vi "FlatToRichni_measurementlink_measurement_v2_GetMetadataResponse.vi"(5 "OutputClusterType":T1, 11 "InputCluster":T11) -> (3 "OutputCluster":T1)   [LabVIEW 2021, in "Measurement Service Client V2.lvlib"]
uses:
  Measurement Service Client V2.lvlib
  ni_measurementlink_measurement_v2_GetMetadataResponse_Flat.ctl
  ni_measurementlink_measurement_v2_MeasurementDetails_Flat.ctl
  ni_measurementlink_measurement_v2_MeasurementSignature_Flat.ctl
  ni_measurementlink_measurement_v2_ConfigurationParameter_Flat.ctl
  google_protobuf_Field_Kind.ctl
  ni_measurementlink_measurement_v2_ConfigurationParameter_AnnotationsEntry_Flat.ctl
  google_protobuf_Any_Flat.ctl
  ni_measurementlink_measurement_v2_Output_Flat.ctl
  ni_measurementlink_measurement_v2_Output_AnnotationsEntry_Flat.ctl
  ni_measurementlink_measurement_v2_UserInterfaceDetails_Flat.ctl
  ni_measurementlink_measurement_v2_GetMetadataResponse.ctl
  ni_measurementlink_measurement_v2_MeasurementDetails.ctl
  ni_measurementlink_measurement_v2_MeasurementSignature.ctl
  ni_measurementlink_measurement_v2_ConfigurationParameter.ctl
  ni_measurementlink_measurement_v2_ConfigurationParameter_AnnotationsEntry.ctl
  google_protobuf_Any.ctl
  ni_measurementlink_measurement_v2_Output.ctl
  ni_measurementlink_measurement_v2_Output_AnnotationsEntry.ctl
  ni_measurementlink_measurement_v2_UserInterfaceDetails.ctl
  FlatToRichni_measurementlink_measurement_v2_ConfigurationParameter.vi
  FlatToRichgoogle_protobuf_Any.vi
  FlatToRichni_measurementlink_measurement_v2_Output.vi
  FlatToRichni_measurementlink_measurement_v2_ConfigurationParameter_AnnotationsEntry.vi
  FlatToRichni_measurementlink_measurement_v2_Output_AnnotationsEntry.vi
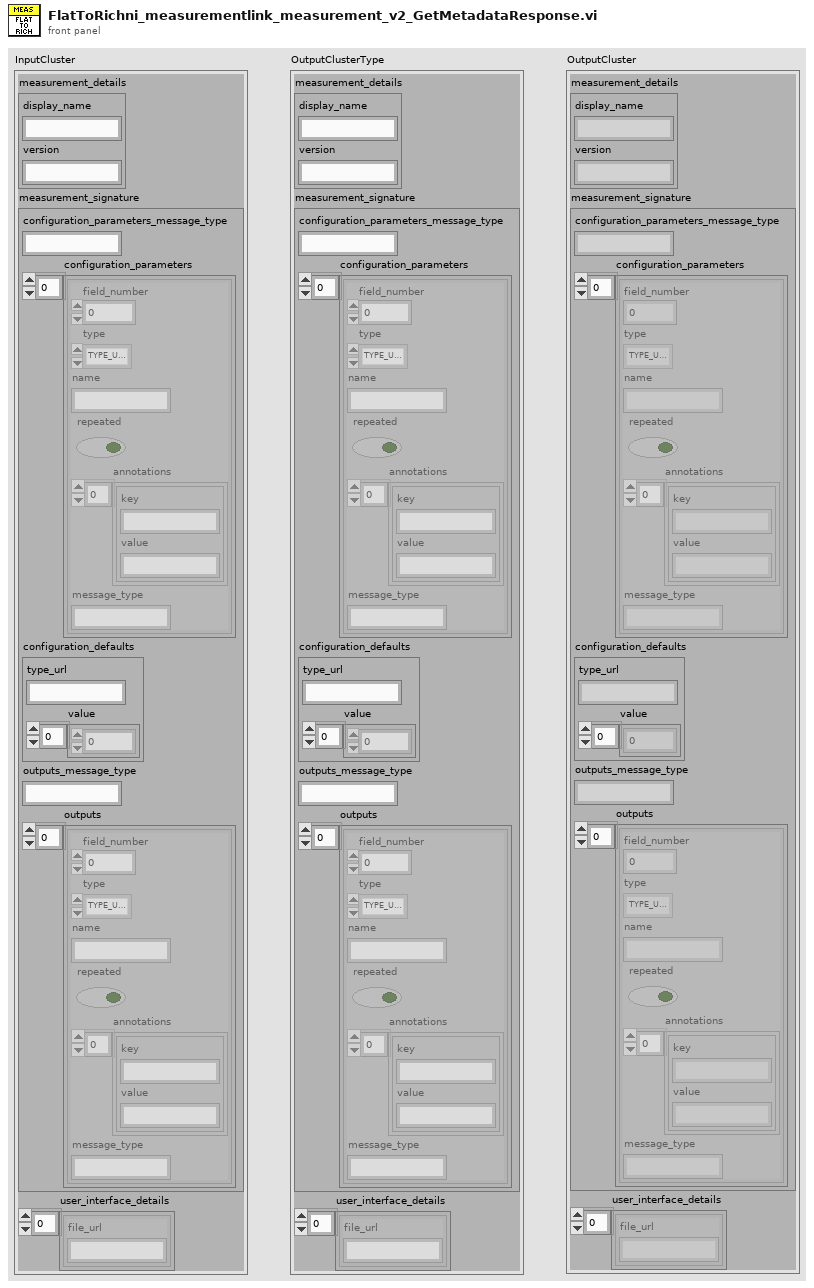
[diagram p1: front panel]
types:
  T1 = typedef "Measurement Service Client V2.lvlib/ni_measurementlink_measurement_v2_GetMetadataResponse.ctl" = cluster{"measurement_details":T2, "measurement_signature":T3, "user_interface_details":T10[]}
  T2 = typedef "Measurement Service Client V2.lvlib/ni_measurementlink_measurement_v2_MeasurementDetails.ctl" = cluster{"display_name":string, "version":string}
  T3 = typedef "Measurement Service Client V2.lvlib/ni_measurementlink_measurement_v2_MeasurementSignature.ctl" = cluster{"configuration_parameters_message_type":string, "configuration_parameters":T4[], "configuration_defaults":T7, "outputs_message_type":string, "outputs":T8[]}
  T4 = typedef "Measurement Service Client V2.lvlib/ni_measurementlink_measurement_v2_ConfigurationParameter.ctl" = cluster{"field_number":i32, "type":T5, "name":string, "repeated":bool, "annotations":T6[], "message_type":string}
  T5 = typedef "Measurement Service Client V2.lvlib/google_protobuf_Field_Kind.ctl" = enum32{"TYPE_UNKNOWN", "TYPE_DOUBLE", "TYPE_FLOAT", "TYPE_INT64", "TYPE_UINT64", "TYPE_INT32", "TYPE_FIXED64", "TYPE_FIXED32", "TYPE_BOOL", "TYPE_STRING", "TYPE_GROUP", "TYPE_MESSAGE", "TYPE_BYTES", "TYPE_UINT32", "TYPE_ENUM", "TYPE_SFIXED32", "TYPE_SFIXED64", "TYPE_SINT32", "TYPE_SINT64"}
  T6 = typedef "Measurement Service Client V2.lvlib/ni_measurementlink_measurement_v2_ConfigurationParameter_AnnotationsEntry.ctl" = cluster{"key":string, "value":string}
  T7 = typedef "Measurement Service Client V2.lvlib/google_protobuf_Any.ctl" = cluster{"type_url":string, "value":u8[]}
  T8 = typedef "Measurement Service Client V2.lvlib/ni_measurementlink_measurement_v2_Output.ctl" = cluster{"field_number":i32, "type":T5, "name":string, "repeated":bool, "annotations":T9[], "message_type":string}
  T9 = typedef "Measurement Service Client V2.lvlib/ni_measurementlink_measurement_v2_Output_AnnotationsEntry.ctl" = cluster{"key":string, "value":string}
  T10 = typedef "Measurement Service Client V2.lvlib/ni_measurementlink_measurement_v2_UserInterfaceDetails.ctl" = cluster{"file_url":string}
  T11 = typedef "Measurement Service Client V2.lvlib/ni_measurementlink_measurement_v2_GetMetadataResponse_Flat.ctl" = cluster{"measurement_details":T12, "measurement_signature":T13, "user_interface_details":T19[]}
  T12 = typedef "Measurement Service Client V2.lvlib/ni_measurementlink_measurement_v2_MeasurementDetails_Flat.ctl" = cluster{"display_name":string, "version":string}
  T13 = typedef "Measurement Service Client V2.lvlib/ni_measurementlink_measurement_v2_MeasurementSignature_Flat.ctl" = cluster{"configuration_parameters_message_type":string, "configuration_parameters":T14[], "configuration_defaults":T16, "outputs_message_type":string, "outputs":T17[]}
  T14 = typedef "Measurement Service Client V2.lvlib/ni_measurementlink_measurement_v2_ConfigurationParameter_Flat.ctl" = cluster{"field_number":i32, "type":T5, "name":string, "repeated":bool, "annotations":T15[], "message_type":string}
  T15 = typedef "Measurement Service Client V2.lvlib/ni_measurementlink_measurement_v2_ConfigurationParameter_AnnotationsEntry_Flat.ctl" = cluster{"key":string, "value":string}
  T16 = typedef "Measurement Service Client V2.lvlib/google_protobuf_Any_Flat.ctl" = cluster{"type_url":string, "value":u8[]}
  T17 = typedef "Measurement Service Client V2.lvlib/ni_measurementlink_measurement_v2_Output_Flat.ctl" = cluster{"field_number":i32, "type":T5, "name":string, "repeated":bool, "annotations":T18[], "message_type":string}
  T18 = typedef "Measurement Service Client V2.lvlib/ni_measurementlink_measurement_v2_Output_AnnotationsEntry_Flat.ctl" = cluster{"key":string, "value":string}
  T19 = typedef "Measurement Service Client V2.lvlib/ni_measurementlink_measurement_v2_UserInterfaceDetails_Flat.ctl" = cluster{"file_url":string}
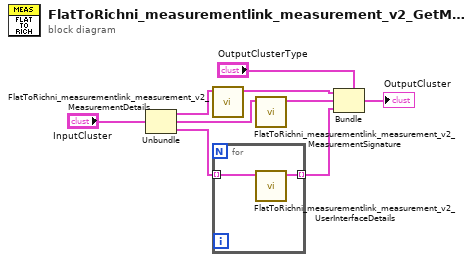
[diagram p0: block diagram]
diagram:
  n1 = Unbundle "Unbundle"("InputCluster") -> ("measurement_details"=w6:T12, "measurement_signature"=w4:T13, "user_interface_details"=w2:T19[])
  n2 = call "FlatToRichni_measurementlink_measurement_v2_MeasurementDetails.vi"("InputCluster"=w6) -> ("OutputCluster"=w5:T2)  [unwired: 10 in]
  n3 = for {
    tunnel: w2 -> [w11] mode=indexing
    tunnel: [w10] -> w1 mode=indexing
    n4 = call "FlatToRichni_measurementlink_measurement_v2_UserInterfaceDetails.vi"("InputCluster"=w11) -> ("OutputCluster"=w10:T10)  [unwired: 10 in]
  }
  n5 = call "FlatToRichni_measurementlink_measurement_v2_MeasurementSignature.vi"("InputCluster"=w4) -> ("OutputCluster"=w3:T3)  [unwired: 10 in]
  n6 = Bundle "Bundle"(cluster="OutputClusterType", "measurement_details"=w5, "measurement_signature"=w3, "user_interface_details"=w1) -> (→"OutputCluster":T1)
